vi "D1.vi"() -> ()   [LabVIEW 2020]
panel:
  in  "Board":i32[][](array[numeric])=[[0, 0, 0, 0], [0, 0, 0, 0], [0, 0, 0, 0], [0, 0, 0, 0]]
  out "Tiles":refnum<vi>[][](array[refnum])
  in  "Title 16":bool
  in  "Title 15":bool
  in  "Title 14":bool
  in  "Title 13":bool
  in  "Title 12":bool
  in  "Title 11":bool
  in  "Title 10":bool
  in  "Title 9":bool
  in  "Title 8":bool
  in  "Title 7":bool
  in  "Title 6":bool
  in  "Title 5":bool
  in  "Title 4":bool
  in  "Title 3":bool
  in  "Title 2":bool
  in  "Title 1":bool
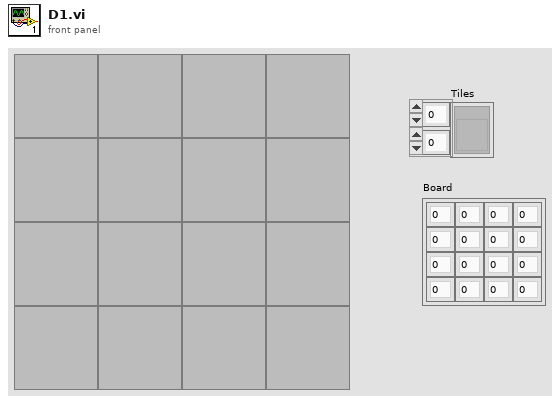
[diagram p1: front panel]
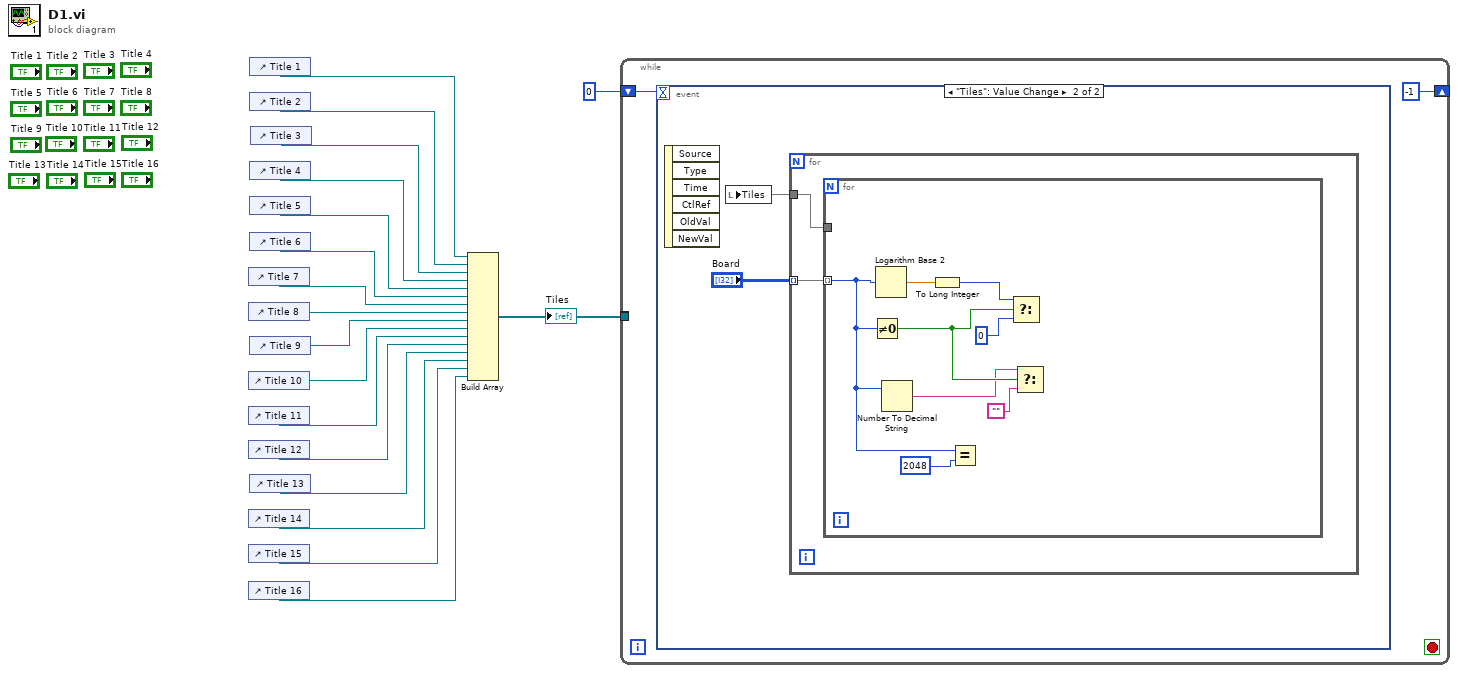
[diagram p0: block diagram]
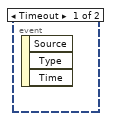
[diagram p2: hidden frame]
diagram:
  n1 = control-ref of="Title 7"() -> (w12:refnum<vi>)
  n2 = control-ref of="Title 8"() -> (w11:refnum<vi>)
  n3 = control-ref of="Title 10"() -> (w9:refnum<vi>)
  n4 = control-ref of="Title 11"() -> (w8:refnum<vi>)
  n5 = control-ref of="Title 12"() -> (w7:refnum<vi>)
  n6 = control-ref of="Title 14"() -> (w5:refnum<vi>)
  n7 = control-ref of="Title 15"() -> (w4:refnum<vi>)
  n8 = control-ref of="Title 16"() -> (w3:refnum<vi>)
  n9 = control-ref of="Title 1"() -> (w18:refnum<vi>)
  n10 = control-ref of="Title 2"() -> (w17:refnum<vi>)
  n11 = control-ref of="Title 4"() -> (w15:refnum<vi>)
  n12 = control-ref of="Title 5"() -> (w14:refnum<vi>)
  n13 = control-ref of="Title 6"() -> (w13:refnum<vi>)
  n14 = control-ref of="Title 9"() -> (w10:refnum<vi>)
  n15 = control-ref of="Title 13"() -> (w6:refnum<vi>)
  n16 = control-ref of="Title 3"() -> (w16:refnum<vi>)
  n17 = Build Array(w18, w17, w16, w15, w14, w13, w12, w11, w10, w9, w8, w7, w6, w5, w4, w3) -> (w2:refnum<vi>[])
  "Tiles" <- w2
  n18 = while {
    tunnel: [w21] -> _
    tunnel: w2 -> [w21]
    shift-right: [-1] -> _
    shift-left: 0 -> [w19]
    stop <- _ stop-if-true
    n19 = event shown="[1] \"Tiles\": Value Change" {
      selector: _ -> [_ _]
      dyn-events: _ -> [_ _]
      timeout: w19 -> [_ _]
      event Timeout {
        n20 = event-data() -> ()  [unwired: 1 in, 3 out]
      }
      event "Tiles": Value Change {
        n21 = event-data() -> ()  [unwired: 1 in, 6 out]
        n22 = for {
          tunnel: [w25] -> w23
          tunnel: "Board" -> [w24] mode=indexing
          n23 = for {
            tunnel: [_] -> w25
            tunnel: w24 -> [w27] mode=indexing
            n24 = Not Equal To 0?(x=w27) -> (x != 0?=w30:bool)
            n25 = Logarithm Base 2(1:w27) -> (0:w33:dbl)
            n26 = Number To Decimal String(number=w27) -> (decimal integer string=w29:string)  [unwired: 1 in]
            n27 = To Long Integer(number=w33) -> (32bit integer=w32:i32)
            n28 = Equal?(x=w27, y=2048) -> ()  [unwired: 1 out]
            n29 = Select(t=w32, s=w30, f=0) -> ()  [unwired: 1 out]
            n30 = Select(t=w29, s=w30, f="") -> ()  [unwired: 1 out]
          }
        }
        n31 = local write "Tiles"(w23) -> ()
      }
    }
  }
